vi "Qwiic.vi"() -> ()   [LabVIEW 2016]
uses:
  VIs/uPythonX/uPythonX.xctl
panel:
  in  "Tab Control":enum32{"Joystick"}(tab)
  in  "Joystick":T1(xcontrol)={"VISA Refnum in"="ASRL23::INSTR", "Python Code"="#https://github.com/sparkfunX/Qwiic_Joystiic\n\nimport machine,utime\n\ni2c = machine.I2C(2)\ni2c.scan()\n#should see an 32 (0x20)\n\nwhile True:\n      data = bytearray(i2c.readfrom_mem(32,0,2))\n      Hpos = data[0]*256 + data[1]\n      utime.sleep_ms(10)\n      data = bytearray(i2c.readfrom_mem(32,2,2))\n      Vpos = data[0]*256 + data[1]\n      utime.sleep_ms(10)\n      data = bytearray(i2c.readfrom_mem(32,4,1))\n      Btn = data[0]\n      print( 'H: %4d   V:%4d   Btn %2d' % (Hpos,Vpos,Btn))\n      utime.sleep_ms(200)\n"}
  in  "Tab Control 2":enum32{"Page 1", "Page 2"}(tab)
  # "B"
  # "R"
  # "B - SCL"
  # "Y - SDA"
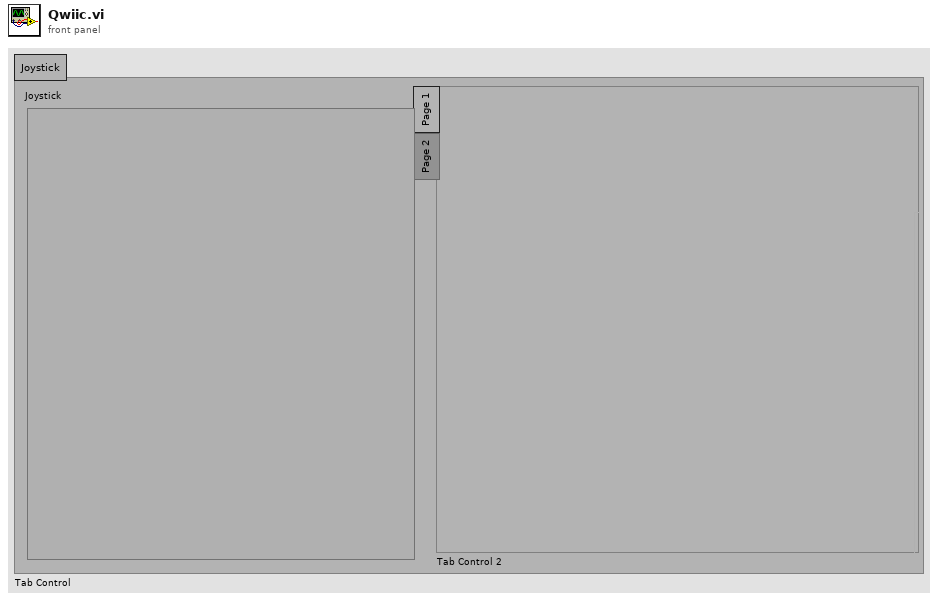
[diagram p1: front panel]
types:
  T1 = cluster{"VISA Refnum in":refnum<visa-resource-name>, "Python Code":string}
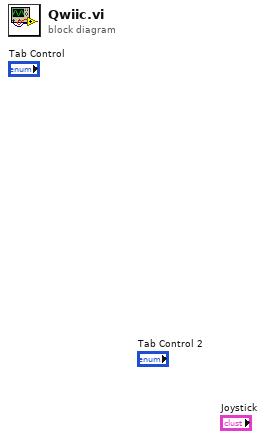
[diagram p0: block diagram]
diagram:
